vi "Notify Subscribers.vi"(8 "error in (no error)":errorcluster, 10 "PublishRequest":refnum<class "PublishRequest.lvclass">, 11 "Topic in":refnum<class "Topic.lvclass">) -> (0 "error out":errorcluster, 3 "Topic out":refnum<class "Topic.lvclass">)   [LabVIEW 2015, in "Mediator.lvlib" / "Topic.lvclass"]
doc: "<License>\nCopyright © 2017 Composed Systems, LLC | All rights reserved\nwww.composed.io\n\nAuthor: Ethan Stern <ethan.stern@composed.io>\n\nThis software is provided \"AS IS\" WITHOUT WARRANTIES, either express or implied, AND IS FOR EDUCATIONAL PURPOSES ONLY.\n</License>"
uses:
  Topic.lvclass
  IMediator/PublishRequest/PublishRequest.lvclass
  Topic.lvclass/Topic.ctl
  IMediator/PublishRequest/PublishRequest.lvclass/PublishRequest.ctl
  IMediator/ISubscriptionPolicy/ISubscriptionPolicy.lvclass/ISubscriptionPolicy.ctl
  IMediator/ISubscriptionPolicy/Read Subscription Policy ID.vi
  <vilib>/Utility/error.llb/Trim Whitespace.vi
  IMediator/ISubscriptionPolicy/ISubscriptionPolicy.lvclass
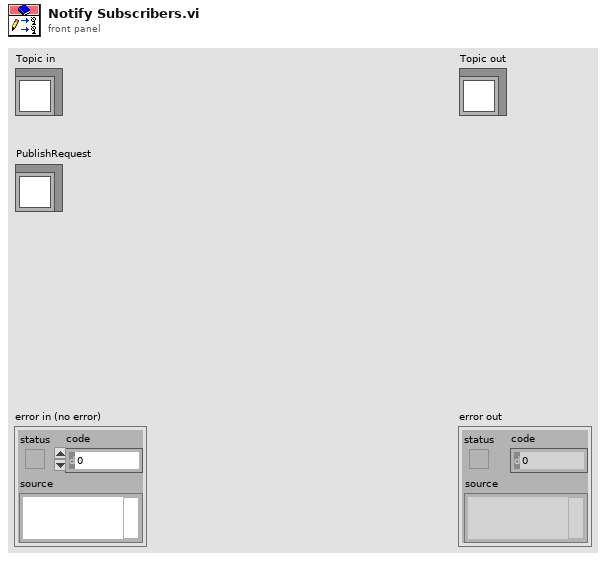
[diagram p1: front panel]
types:
  T1 = typedef "IMediator.lvlib/ISubscriptionPolicy.lvclass/ISubscriptionPolicy Reference.ctl" = refnum<data-value>
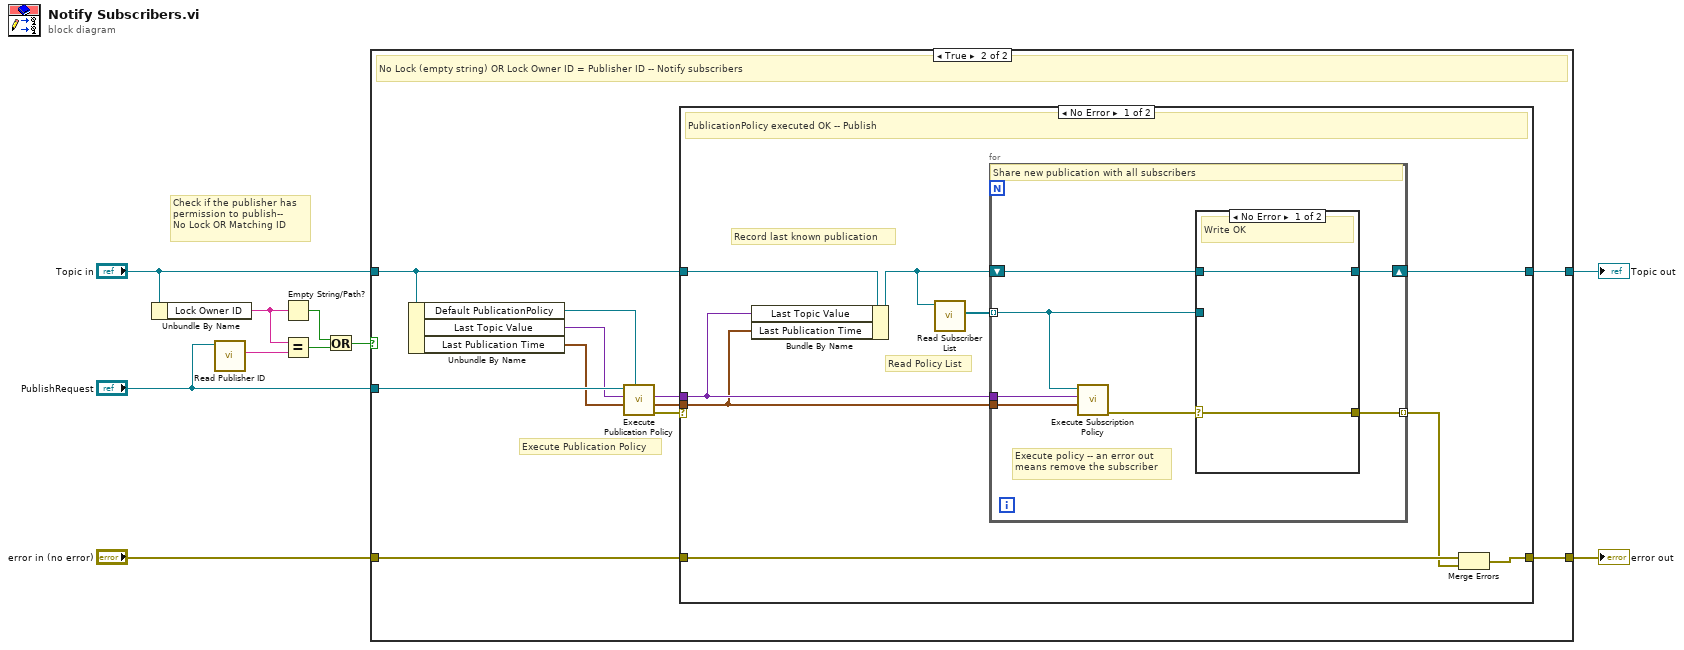
[diagram p0: block diagram]
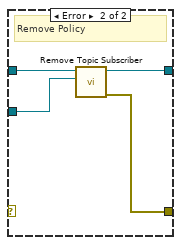
[diagram p3: hidden frame]
diagram:
  # "Check if the publisher has\npermission to publish--\nNo Lock OR Matching ID"
  n1 = Unbundle By Name("Topic in") -> ("Lock Owner ID"=w6:string)
  n2 = call "Read Publisher ID.vi"("PublishRequest In"="PublishRequest") -> ("Publisher ID"=w1:string)  [unwired: 10 in]
  n3 = Empty String/Path?(string/path=w6) -> (empty?=w5:bool)
  n4 = Equal?(x=w6, y=w1) -> (x = y?=w4:bool)
  n5 = Or(x=w5, y=w4) -> (x .or. y?=w3:bool)
  n6 = case shown="True" w3 {
    tunnel: "error in (no error)" -> [w12 w23]
    tunnel: [w12 w22] -> w9
    tunnel: [w11 w21] -> w8
    tunnel: "Topic in" -> [w11 w19]
    tunnel: "PublishRequest" -> [_ w20]
    frame False {
      # "This publication was not from the lock holder -- Ignore it"
    }
    frame True {
      # "Execute Publication Policy"
      # "No Lock (empty string) OR Lock Owner ID = Publisher ID -- Notify subscribers"
      n7 = Unbundle By Name(w19) -> ("Default PublicationPolicy"=w18:refnum<class "IPublicationPolicy.lvclass">, "Last Topic Value"=w17:variant, "Last Publication Time"=w16:timestamp)
      n8 = call-dynamic "Execute Publication Policy.vi"("Default PublicationPolicy"=w18, "Last Publish Time"=w16, "Last Published Value"=w17, "PublishRequest"=w20) -> ("error out"=w14:errorcluster, "Publication Time"=w13:timestamp, "Value to Publish"=w15:variant)  [unwired: 5 in]
      n9 = case shown="No Error" w14 {
        tunnel: w23 -> [w32 w47]
        tunnel: [w31 w47] -> w22
        tunnel: [w29 w46] -> w21
        tunnel: w19 -> [w26 w46]
        tunnel: w15 -> [w25 _]
        tunnel: w13 -> [w24 _]
        frame No Error {
          # "Read Policy List"
          # "Record last known publication"
          # "PublicationPolicy executed OK -- Publish"
          n10 = Bundle By Name(cluster=w26, "Last Topic Value"=w25, "Last Publication Time"=w24) -> (w27:refnum<class "Topic.lvclass">)
          n11 = call "Read Subscriber List.vi"("Topic in"=w27) -> ("Subscriber Policy List"=w28:T1[])  [unwired: 10 in]
          n12 = for {
            tunnel: w28 -> [w33] mode=indexing
            tunnel: w25 -> [w38]
            tunnel: [w39] -> w30 mode=indexing
            tunnel: w24 -> [w34]
            shift-right: [w36] -> w29
            shift-left: w27 -> [w37]
            # "Execute policy -- an error out\nmeans remove the subscriber"
            # "Share new publication with all subscribers"
            n13 = call "Execute Subscription Policy.vi"("Publish Time"=w34, "New Topic Value"=w38, "Subscription Policy"=w33) -> ("error out (Unsubscribe?)"=w35:errorcluster)  [unwired: 8 in]
            n14 = case shown="No Error" w35 {
              selector: w35 -> [w40 _]
              tunnel: [w40 w45] -> w39
              tunnel: w37 -> [w41 w44]
              tunnel: [w41 w43] -> w36
              tunnel: w33 -> [_ w42]
              frame No Error {
                # "Write OK"
              }
              frame Error {
                # "Remove Policy"
                n15 = call "Remove Topic Subscriber.vi"("Subscription Policy"=w42, "Topic in"=w44) -> ("error out"=w45:errorcluster, "Topic out"=w43:refnum<class "Topic.lvclass">)  [unwired: 8 in]
              }
            }
          }
          n16 = Merge Errors(w32, w30) -> (w31:errorcluster)
        }
        frame Error {
          # "Error executing PublicationPolicy -- Do not publish"
        }
      }
    }
  }
  "error out" <- w9
  "Topic out" <- w8
